vi "Error Loop.vi"   [LabVIEW 2013]
uses:
  <vilib>/Utility/file.llb/Write To Spreadsheet File (string).vi
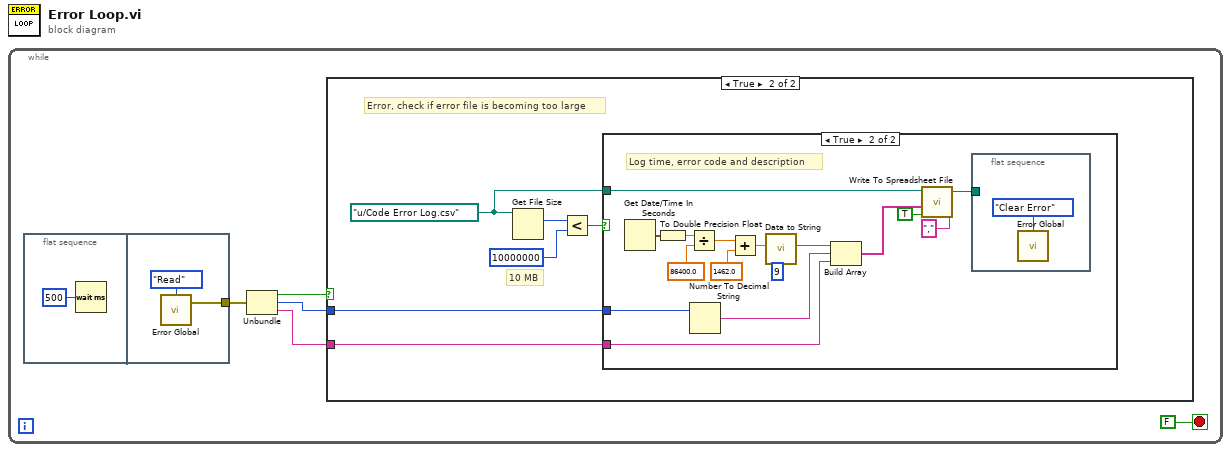
[diagram p0: block diagram]
diagram:
  n1 = while {
    stop <- FALSE stop-if-true
    n2 = flat-sequence {
      tunnel: [w30] -> w4
      frame #0 {
        n3 = Wait (ms)(milliseconds to wait=u32 500) -> ()  [unwired: 1 out]
      }
      frame #1 {
        n4 = call "Error Global.vi"("Mode"=enum16{"Read", "Write", "Clear Error"}."Read") -> ("Error Out"=w30:errorcluster)  [unwired: 4 in]
      }
    }
    n5 = Unbundle(w4) -> ("status"=w3:bool, "code"=w2:i32, "source"=w1:string)
    n6 = case shown="True" w3 {
      tunnel: w2 -> [_ w7]
      tunnel: w1 -> [_ w6]
      frame False {
        # "No error, no action"
      }
      frame True {
        w8 = path "u:/Code Error Log.csv" ("Fuel Log Path")
        # "10 MB"
        # "Error, check if error file is becoming too large"
        n7 = Get File Size(file=w8) -> (size (in bytes)=w11:i64)  [unwired: 1 in, 2 out]
        n8 = Less?(x=w11, y=i64 10000000 ("size (in bytes)")) -> (x < y?=w9:bool)
        n9 = case shown="True" w9 {
          tunnel: w8 -> [_ w16]
          tunnel: w7 -> [_ w27]
          tunnel: w6 -> [_ w25]
          frame False {
            # "File at specified capacity\nno more error logging"
          }
          frame True {
            # "Log time, error code and description"
            n10 = Get Date/Time In Seconds() -> (seconds since 1Jan1904=w23:timestamp)
            n11 = To Double Precision Float(number=w23) -> (double precision float=w24:dbl)
            n12 = Divide(x=w24, y=86400.0) -> (x/y=w20:dbl)
            n13 = Number To Decimal String(number=w27) -> (decimal integer string=w26:string)  [unwired: 1 in]
            n14 = Add(x=w20, y=1462.0) -> (x+y=w19:dbl)
            n15 = call "Data to String.vi"("Precision (2)"=i16 9, "Data"=w19) -> ("String Data"=w17:string)  [unwired: 9 in]
            n16 = Build Array(w17, w26, w25) -> (w14:string[])
            n17 = call-poly <vilib>:"Write To Spreadsheet File.vi"("delimiter (\\t)"="," ("delimiter (\\t)"), "append to file? (new file:F)"=TRUE, "1D data"=w14, "file path (dialog if empty)"=w16) -> ("new file path (Not A Path if cancelled)"=w12:path)  [unwired: 4 in]
            n18 = flat-sequence {
              tunnel: w12 -> [_]
              frame #0 {
                n19 = call "Error Global.vi"("Mode"=enum16{"Read", "Write", "Clear Error"}."Clear Error") -> ()  [unwired: 4 in, 1 out]
              }
            }
          }
        }
      }
    }
  }
